vi "Configure.vi"(8 "error in (no error)":errorcluster, 11 "Stage_MadCityLab in":refnum<class "Stage_MadCityLab.lvclass">) -> (0 "error out":errorcluster, 3 "Stage_MadCityLab out":refnum<class "Stage_MadCityLab.lvclass">)   [LabVIEW 2020, in "Stage_MadCityLab.lvlib" / "Stage_MadCityLab.lvclass"]
uses:
  Stage_MadCityLab.lvclass
  Hardware Abstraction Layer/Component/Stage/Stage/Stage.lvclass
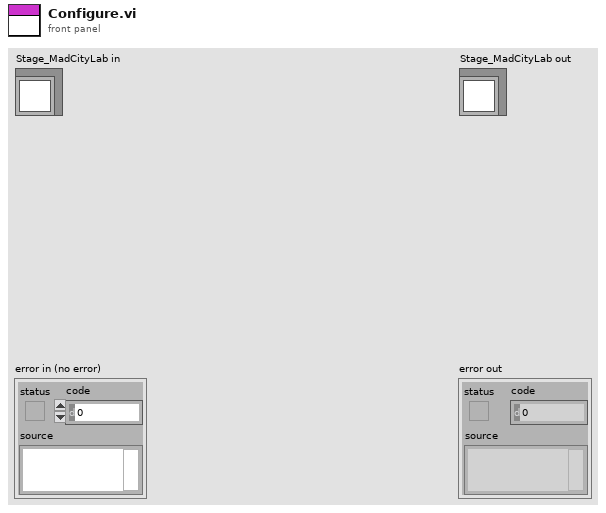
[diagram p1: front panel]
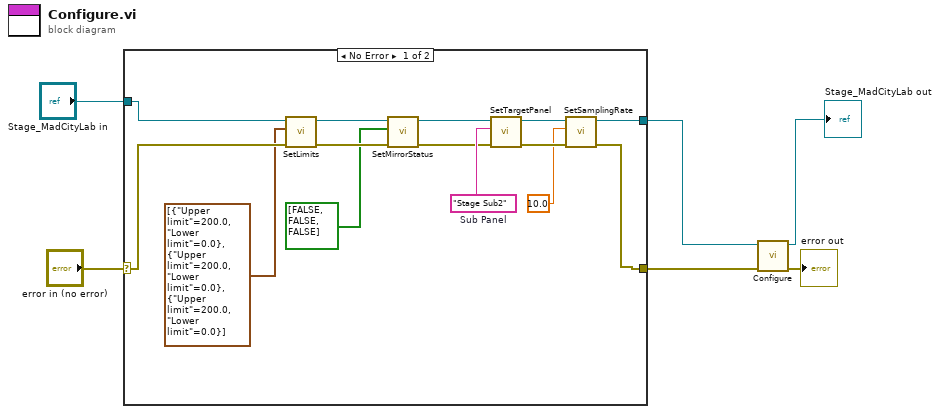
[diagram p0: block diagram]
diagram:
  n1 = case shown="No Error" "error in (no error)" {
    selector: "error in (no error)" -> [w19 w22]
    tunnel: [w14 w22] -> w3
    tunnel: [w12 w21] -> w1
    tunnel: "Stage_MadCityLab in" -> [w20 w21]
    frame No Error {
      w16 = "Stage Sub2"  # Sub Panel
      n2 = call-dynamic "SetLimits.vi"("error in (no error)"=w19, "Limits"=cluster{"Upper limit":dbl, "Lower limit":dbl}[] [{"Upper limit"=200.0, "Lower limit"=0.0}, {"Upper limit"=200.0, "Lower limit"=0.0}, {"Upper limit"=200.0, "Lower limit"=0.0}], "Stage in"=w20) -> ("error out"=w17:errorcluster, "Stage out"=w9:refnum<class "Stage_MadCityLab.lvclass">)  [unwired: 7 in]
      n3 = call-dynamic "SetMirrorStatus.vi"("error in (no error)"=w17, "Mirror"=bool[] [FALSE, FALSE, FALSE], "Stage in"=w9) -> ("error out"=w10:errorcluster, "Stage out"=w8:refnum<class "Stage_MadCityLab.lvclass">)  [unwired: 7 in]
      n4 = call-dynamic "SetTargetPanel.vi"("error in (no error)"=w10, "TargetPanel"=w16, "GRMActor in"=w8) -> ("error out"=w15:errorcluster, "GRMActor out"=w13:refnum<class "Stage_MadCityLab.lvclass">)  [unwired: 7 in]
      n5 = call-dynamic "SetSamplingRate.vi"("error in (no error)"=w15, "SamplingRate(Hz)"=10.0 ("Interval(ms)"), "Device in"=w13) -> ("error out"=w14:errorcluster, "Device out"=w12:refnum<class "Stage_MadCityLab.lvclass">)  [unwired: 7 in]
    }
    frame Error {
    }
  }
  n6 = call-parent "Configure.vi"("error in (no error)"=w3, "Device in"=w1) -> ("error out"=→"error out":errorcluster, "Device out"=→"Stage_MadCityLab out":refnum<class "Stage_MadCityLab.lvclass">)  [unwired: 8 in]
